vi "Q8381 QRY Level scale.vi"(2 "GPIB address":u16=8 max=31 step=1, 3 "VISA resource name":refnum<visa-resource-name>) -> (0 "Level value":sgl format="%.2f", 1 "GPIB status":bool)   [LabVIEW 2017]
panel:
  out "Level data":string
  out "Program code":string
  # "Query level scale"
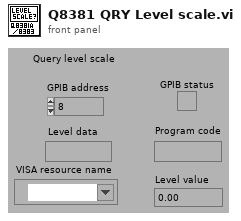
[diagram p1: front panel]
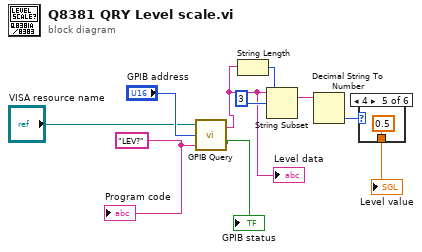
[diagram p0: block diagram]
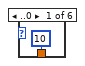
[diagram p2: hidden frame]
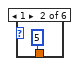
[diagram p3: hidden frame]
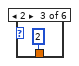
[diagram p4: hidden frame]
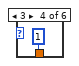
[diagram p5: hidden frame]
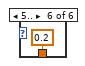
[diagram p6: hidden frame]
diagram:
  w2 = "LEV?"
  n1 = call "GPIB Query.vi"("Command String"=w2, "Address"="GPIB address", "VISA resource name"="VISA resource name") -> ("Error"=→"GPIB status":bool, "Query Data"=w4:string)
  "Level data" <- w4
  n2 = String Length(string=w4) -> (length=w10:i32)
  n3 = String Subset(string=w4, offset (0)=3, length (rest)=w10) -> (substring=w7:string)
  n4 = Decimal String To Number(string=w7) -> (number=w6:i32)  [unwired: 2 in, 1 out]
  n5 = case shown="4" w6 {
    tunnel: [10 5 2 1 0.5 0.2] -> w8
    frame ..0 {
    }
    frame 1 {
    }
    frame 2 {
    }
    frame 3 {
    }
    frame 4 {
    }
    frame 5.. {
    }
  }
  "Level value" <- w8
  "Program code" <- w2
